vi "Paths Sub-Parser.vi"(0 "XML File Path In":path, 2 "error in (no error)":errorcluster) -> (3 "XML File Path Out":path, 4 "paths":T1[](array[typedef]), 5 "funnels":T3[](array[typedef]), 6 "error out":errorcluster)   [LabVIEW 2019]
doc: "This VI takes an array of XML path nodes as input and uses LabVIEW's built-in XPath parser to pull out information about each path. Specifically, it gets the style ('style') and the path data ('d') and parses each one. Then it determines whether the path is actually a funnel and creates two arrays accordingly."
uses:
  typedefs/Parsed Funnel - Cluster.ctl
  <vilib>/Analysis/Matrix/Datatypes/RealMatrix.ctl
  typedefs/Parsed Path - Cluster.ctl
  <vilib>/Analysis/baseanly.llb/Real A x B.vi
  <vilib>/Analysis/NI_AALBase.lvlib
  <vilib>/Analysis/Matrix/NI_Matrix.lvlib
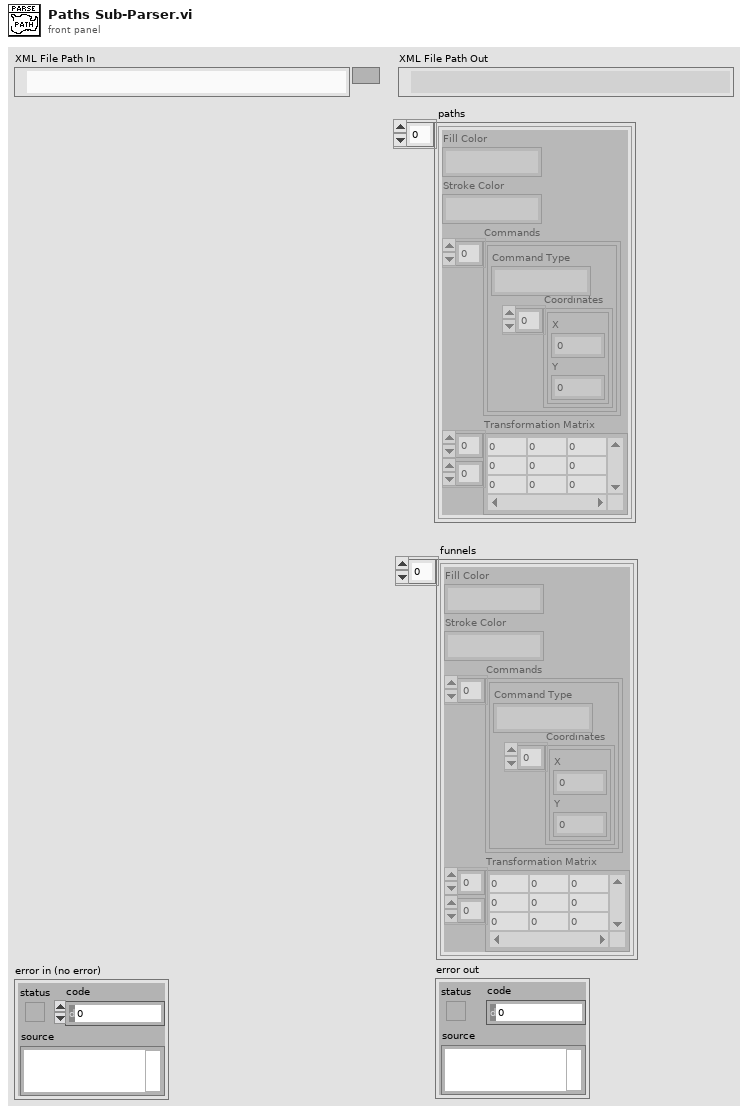
[diagram p1: front panel]
types:
  T1 = typedef "Parsed Path - Cluster.ctl" = cluster{"Fill Color":string, "Stroke Color":string, "Commands":cluster{"Command Type":string, "Coordinates":cluster{"X":dbl, "Y":dbl}[]}[], "Transformation Matrix":T2}
  T2 = typedef "NI_Matrix.lvlib/RealMatrix.ctl" = dbl[][]
  T3 = typedef "Parsed Funnel - Cluster.ctl" = cluster{"Fill Color":string, "Stroke Color":string, "Commands":cluster{"Command Type":string, "Coordinates":cluster{"X":dbl, "Y":dbl}[]}[], "Transformation Matrix":T2}
  T4 = cluster{"Command Type":string, "Coordinates":cluster{"X":dbl, "Y":dbl}[]}[]
  T5 = cluster{"Fill":string, "Stroke":string, "Commands":cluster{"Command Type":string, "Coordinates":cluster{"X":dbl, "Y":dbl}[]}[], "Transformation Matrix":T2}
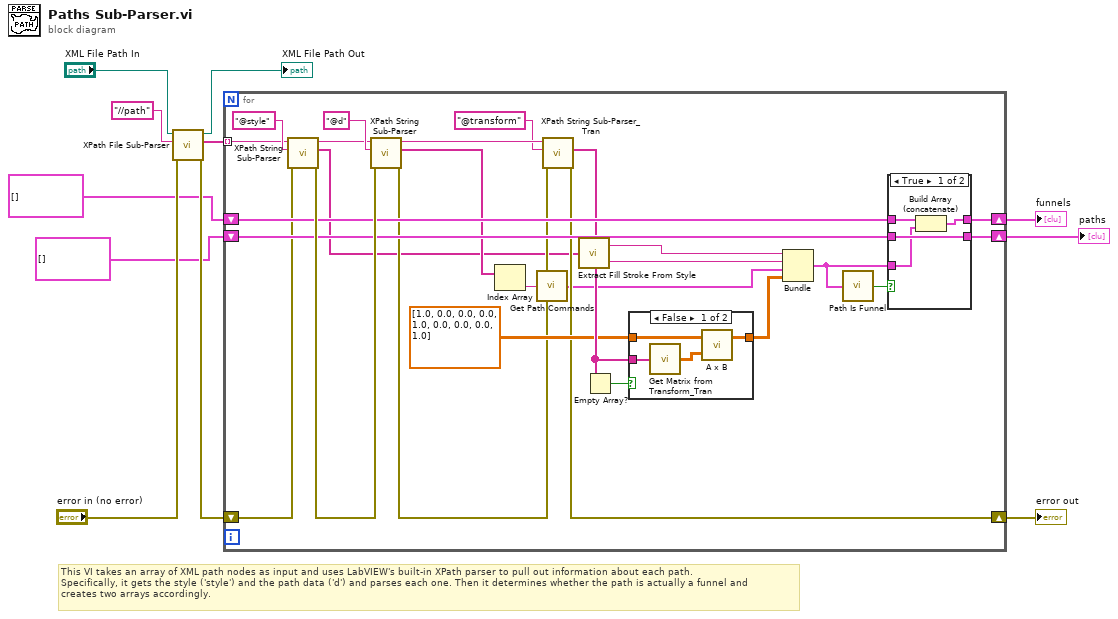
[diagram p0: block diagram]
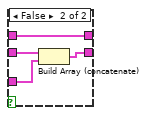
[diagram p3: hidden frame]
diagram:
  # "This VI takes an array of XML path nodes as input and uses LabVIEW's built-in XPath parser to pull out information about each path. \nSpecifically, it gets the style ('style') and the path data ('d') and parses each one. Then it determines whether the path is actually a funnel and\ncreates two arrays accordingly."
  n1 = call "XPath File Sub-Parser.vi"("error in (no error)"="error in (no error)", "XPath Expression"="//path" ("XPath expression"), "XML File Path In"="XML File Path In") -> ("error out"=w3:errorcluster, "Array of Results"=w8:string[], "XML File Path Out"=→"XML File Path Out":path)  [unwired: 6 in]
  n2 = for {
    tunnel: w8 -> [w34] mode=indexing
    shift-right: [w17] -> w11
    shift-left: w3 -> [w15]
    shift-right: [w28] -> w10
    shift-left: T1[] [] -> [w30]
    shift-right: [w27] -> w5
    shift-left: T3[] [] -> [w29]
    n3 = call "XPath String Sub-Parser.vi"("error in (no error)"=w15, "XPath expression"="@style", "XML String In"=w34) -> ("error out"=w36:errorcluster, "Array of Results"=w12:string[], "XML String Out"=w31:string)  [unwired: 6 in]
    n4 = call "XPath String Sub-Parser.vi"("error in (no error)"=w36, "XPath expression"="@d", "XML String In"=w31) -> ("error out"=w18:errorcluster, "Array of Results"=w21:string[], "XML String Out"=w19:string)  [unwired: 6 in]
    n5 = Index Array(array=w21) -> (element=w13:string)  [unwired: 1 in]
    n6 = call "Get Path Commands.vi"("Commands Raw Data"=w13) -> ("Commands"=w14:T4)
    n7 = call "XPath String Sub-Parser_Tran.vi"("error in (no error)"=w18, "XPath expression"="@transform", "XML String"=w19) -> ("error out"=w17:errorcluster, "Array of Results"=w22:string[])  [unwired: 6 in, 1 out]
    n8 = call "Extract Fill Stroke From Style.vi"("Array of Results"=w12) -> ("Fill"=w32:string, "Stroke"=w33:string)
    n9 = Empty Array?(array=w22) -> (empty?=w26:bool)
    n10 = case shown="False" w26 {
      tunnel: [w41 w42] -> w23
      tunnel: w22 -> [w40 _]
      tunnel: T2 [[1.0, 0.0, 0.0], [0.0, 1.0, 0.0], [0.0, 0.0, 1.0]] ("Transformation Matrix") -> [w39 w42]
      frame False {
        n11 = call "Get Matrix from Transform_Tran.vi"("Transform Attributes"=w40) -> ("Matrix"=w38:T2)
        n12 = call-poly <vilib>:"A x B.vi"("B"=w38, "A"=w39) -> ("A x B"=w41:T2)  [unwired: 1 out]
      }
      frame True {
      }
    }
    n13 = Bundle("Fill"=w32, "Stroke"=w33, "Commands"=w14, "Transformation Matrix"=w23) -> (w24:T5)  [unwired: 1 in]
    n14 = call "Path Is Funnel.vi"("Path Information"=w24) -> ("Is Funnel?"=w25:bool)
    n15 = case shown="True" w25 {
      tunnel: w30 -> [w46 w48]
      tunnel: w29 -> [w45 w50]
      tunnel: [w46 w47] -> w28
      tunnel: w24 -> [w44 w49]
      tunnel: [w43 w50] -> w27
      frame True {
        n16 = Build Array (concatenate)(w45, w44) -> (w43:T3[])
      }
      frame False {
        n17 = Build Array (concatenate)(w48, w49) -> (w47:T1[])
      }
    }
  }
  "error out" <- w11
  "funnels" <- w5
  "paths" <- w10
